vi "PostUserInterfaceRefnum.vi"(8 "error in (no error)":errorcluster, 9 "VI Refnum":refnum<vi>, 10 "Panel":string, 11 "Device in":refnum<class "Device.lvclass">) -> (0 "error out":errorcluster, 3 "Device out":refnum<class "Device.lvclass">)   [LabVIEW 2020, in "Device.lvlib" / "Device.lvclass"]
uses:
  Device.lvclass
  C:/Program Files/National Instruments/LabVIEW 2020/vi.lib/ActorFramework/Actor/Actor.lvclass
  <vilib>/ActorFramework/Actor/Actor.lvclass/Actor.ctl
  Interface/DockStation Messages/InsertDevicePanel Msg/InsertDevicePanel Msg.lvclass/InsertDevicePanel Msg.ctl
  <vilib>/ActorFramework/Message Enqueuer/Message Enqueuer.lvclass/Message Enqueuer.ctl
  <vilib>/ActorFramework/Message Enqueuer/Enqueue.vi
  Interface/DockStation Messages/InsertDevicePanel Msg/InsertDevicePanel Msg.lvclass
  C:/Program Files/National Instruments/LabVIEW 2020/vi.lib/ActorFramework/Message/Message.lvclass
  <vilib>/ActorFramework/Message Priority Queue/Priority Enqueue.vi
  <vilib>/ActorFramework/Actor/Actor.lvclass
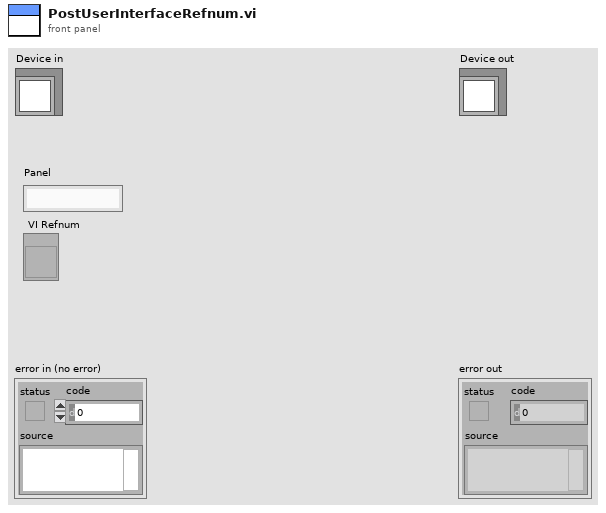
[diagram p1: front panel]
types:
  T1 = enum32{"Invalid", "Standard", "Closed", "Hidden", "Minimized", "Maximized"}
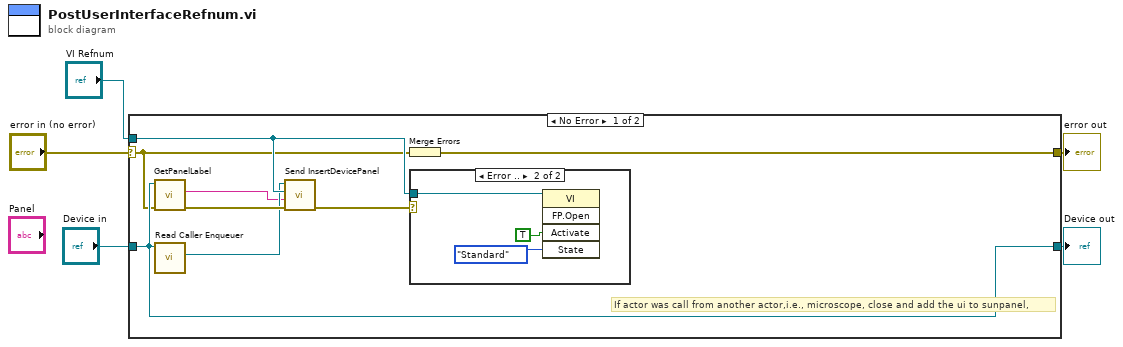
[diagram p0: block diagram]
diagram:
  n1 = case shown="No Error" "error in (no error)" {
    selector: "error in (no error)" -> [w10 w18]
    tunnel: [w13 w18] -> w4
    tunnel: [w11 w17] -> w3
    tunnel: "Device in" -> [w11 w17]
    tunnel: "VI Refnum" -> [w12 _]
    frame No Error {
      # "If actor was call from another actor,i.e., microscope, close and add the ui to sunpanel,"
      n2 = call-dynamic "GetPanelLabel.vi"("error in (no error)"=w10, "Device in"=w11) -> ("error out"=w9:errorcluster, "Sub Panel"=w6:string)  [unwired: 7 in, 1 out]
      n3 = call <vilib>:"Read Caller Enqueuer.vi"("Actor"=w11) -> ("Caller Enqueuer"=w8:refnum<class "Message Enqueuer.lvclass">)  [unwired: 10 in]
      n4 = call "Send InsertDevicePanel.vi"("error in (no error)"=w9, "Panel"=w6, "VI Refnum"=w12, "Message Enqueuer"=w8) -> ("error out"=w7:errorcluster)  [unwired: 6 in, 1 out]
      n5 = Merge Errors(w10) -> (w13:errorcluster)
      n6 = case shown="Error .." w7 {
        tunnel: w12 -> [_ w16]
        frame No Error {
        }
        frame Error {
          n7 = invoke class="VI" method="FP.Open"(reference=w16, "Activate"=TRUE ("Activate?"), "State"=T1."Standard") -> ()  [unwired: 2 in, 5 out]
        }
      }
    }
    frame Error {
    }
  }
  "error out" <- w4
  "Device out" <- w3
